vi "check_piezo_travel.vi"() -> ()   [LabVIEW 2015]
uses:
  <vilib>/DAQmx/create/channels.llb/DAQmx Create Channel (AO-Voltage-Basic).vi
  <vilib>/DAQmx/configure/timing.llb/DAQmx Timing (Sample Clock).vi
  <resource>/objmgr/daqmx.rc
  <vilib>/DAQmx/write.llb/DAQmx Write (Analog 1D DBL 1Chan NSamp).vi
  <vilib>/Analysis/NI_AALBase.lvlib
  <vilib>/Analysis/3filter.llb/Bessel Filter (DBL).vi
  <vilib>/Analysis/3filter.llb/Filter Passband Type.ctl
panel:
  out "error out 2":errorcluster
  out "error out":errorcluster
  out "AO SampClk.Rate":dbl
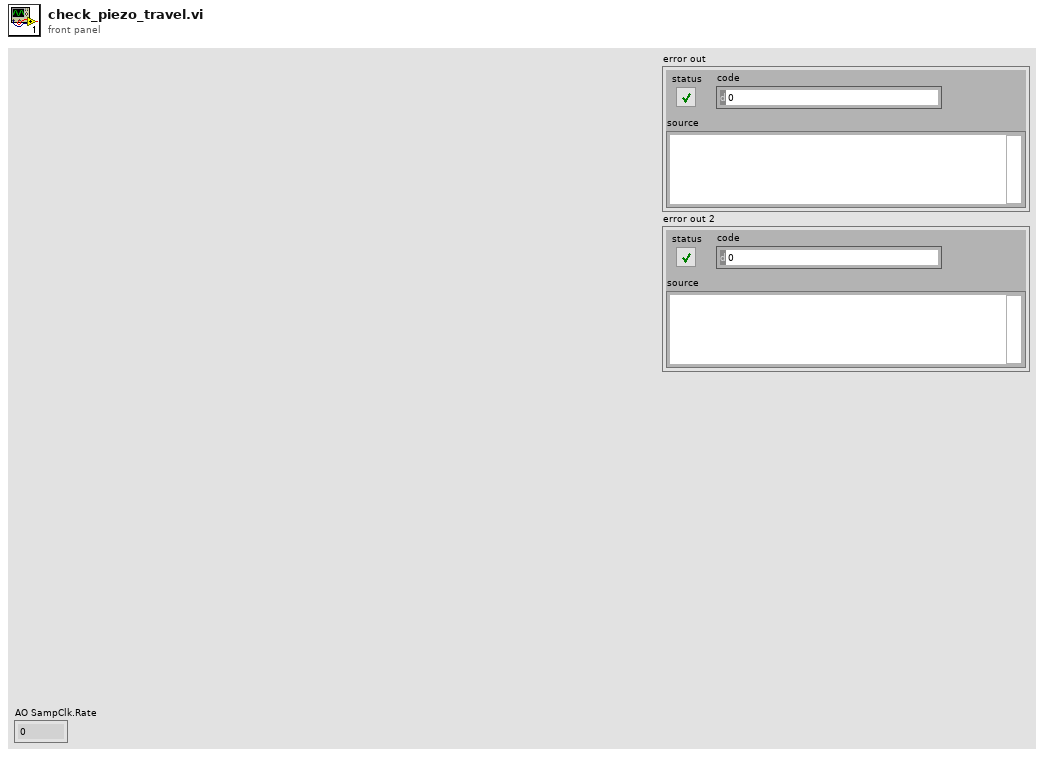
[diagram p1: front panel]
types:
  T1 = typedef "NI_AALBase.lvlib/Filter Passband Type.ctl" = enum32{"Lowpass", "Highpass", "Bandpass", "Bandstop"}
  T2 = typedef "Image Type" = u32
  T3 = typedef "IMAQ Image.ctl" = refnum<image>
  T4 = cluster{"Rows Per Strip":i32, "Photometric":i32, "Compression Type":i32}
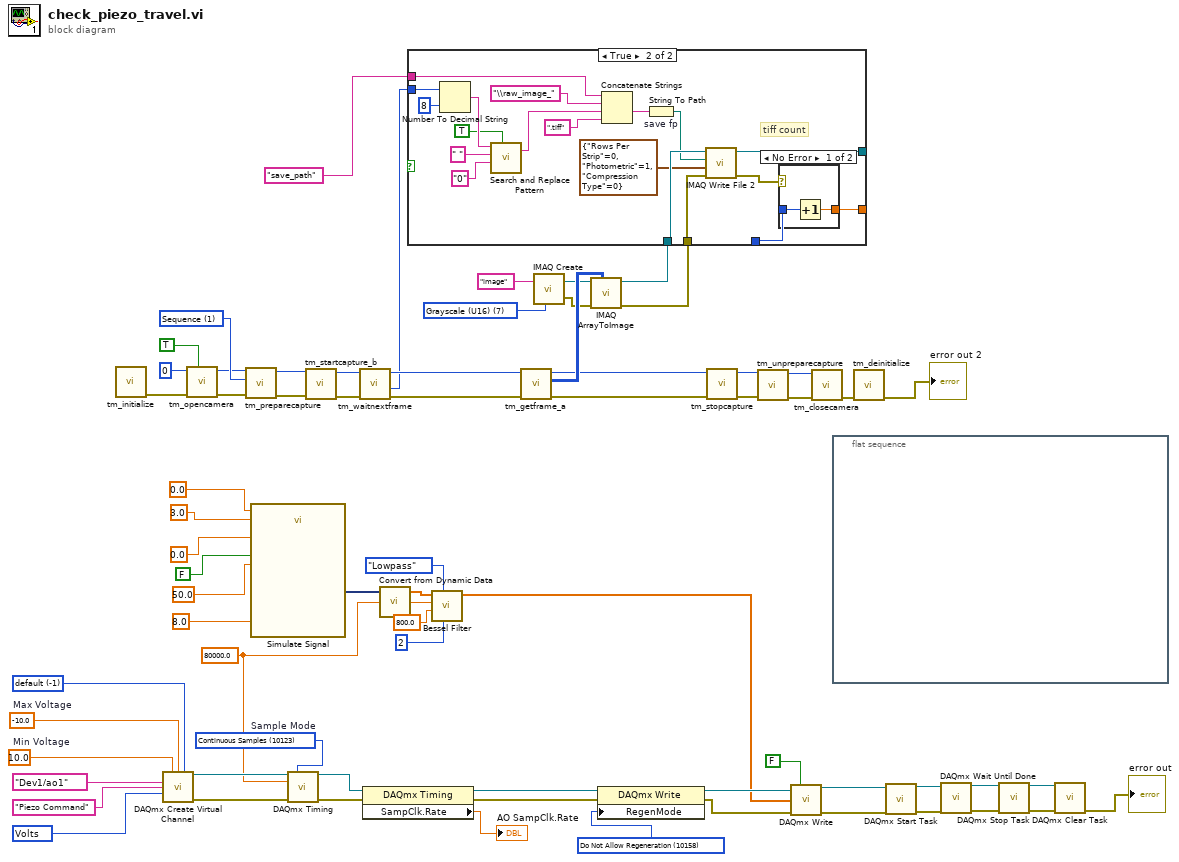
[diagram p0: block diagram]
diagram:
  w10 = 80000.0 ("Rate")
  w34 = 10158 items=["Allow Regeneration"=10097, "Do Not Allow Regeneration"=10158] ("RegenMode")
  w38 = 10123 items=["Finite Samples"=10178, "Continuous Samples"=10123, "Hardware Timed Single Point"=12522]  # Sample Mode
  w45 = -1 items=["default"=-1, "RSE"=10083, "NRSE"=10078, "Differential"=10106, "Pseudodifferential"=12529] ("input terminal configuration")
  w44 = 10348 items=["Volts"=10348, "From Custom Scale"=10065] ("units")
  w41 = 10.0  # Min Voltage
  w42 = -10.0  # Max Voltage
  w57 = T2 7 items=["Grayscale (U8)", "Grayscale (I16)", "Grayscale (SGL)", "Complex (CSG)", "RGB (U32)", "HSL (U32)", "RGB (U64)", "Grayscale (U16)"] ("Image Type")
  w69 = 1 items=["Snap", "Sequence"] ("Capture mode")
  n1 = call <userlib>:"tm_initialize.vi"() -> ("error out"=w68:errorcluster)  [unwired: 8 in, 3 out]
  n2 = call-poly <vilib>:"DAQmx Create Virtual Channel.vi"("maximum value"=w41, "minimum value"=w42, "output terminal configuration"=w45, "physical channels"=tag "Dev1/ao1", "name to assign"="Piezo Command", "units"=w44) -> ("task out"=w39:refnum<k21>, "error out"=w40:errorcluster)  [unwired: 8 in]
  n3 = call <userlib>:"tm_opencamera.vi"("Force Open"=TRUE, "error in (no error)"=w68, "Camera Index"=0) -> ("error out"=w64:errorcluster, "Handle out"=w65:u32)  [unwired: 6 in, 1 out]
  n4 = call <userlib>:"tm_preparecapture.vi"("error in (no error)"=w64, "Capture mode"=w69, "Handle in"=w65) -> ("error out"=w62:errorcluster, "Handle out"=w63:u32)  [unwired: 5 in, 2 out]
  n5 = call "Simulate Signal"("Offset"=0.0, "Duty Cycle (%)"=50.0, "Reset Signal"=FALSE, "Frequency"=3.0, "Amplitude"=8.0, "Phase"=0.0) -> ("Square"=w12:dynamicdata)  [unwired: 8 in, 1 out]
  n6 = call-poly <vilib>:"DAQmx Timing.vi"("task/channels in"=w39, "sample mode"=w38, "rate"=w10, "error in"=w40) -> ("task out"=w36:refnum<k21>, "error out"=w35:errorcluster)  [unwired: 10 in]
  n7 = call <userlib>:"tm_startcapture_b.vi"("error in (no error)"=w62, "Handle in"=w63) -> ("error out"=w60:errorcluster, "Handle out"=w61:u32)  [unwired: 8 in]
  n8 = call <userlib>:"tm_waitnextframe.vi"("error in (no error)"=w60, "Handle in"=w61) -> ("error out"=w58:errorcluster, "Frame Count"=w50:i32, "Handle out"=w59:u32)  [unwired: 6 in, 1 out]
  n9 = property class="DAQmx Timing"(reference=w36, error in=w35) -> (reference out=w47:refnum<k21>, error out=w48:errorcluster, "SampClk.Rate"=→"AO SampClk.Rate":dbl)
  n10 = call "Convert from Dynamic Data"("Dynamic Data Type"=w12) -> ("Array"=w11:dbl[])  [unwired: 3 in]
  n11 = call-poly <vilib>:"Bessel Filter.vi"("order"=2, "filter type"=Filter_Passband_Type."Lowpass", "high cutoff freq: fh"=800.0, "sampling freq: fs"=w10, "X"=w11) -> ("Filtered X"=w2:dbl[])  [unwired: 3 in, 1 out]
  n12 = call <userlib>:"tm_getframe_a.vi"("error in (no error)"=w58, "Handle in"=w59) -> ("error out"=w27:errorcluster, "Data 16"=w55:u16[][], "Handle out"=w28:u32)  [unwired: 5 in, 2 out]
  n13 = call "IMAQ Create"("Image Name"="image", "Image Type"=w57) -> ("New Image"=w53:T3, "error out"=w52:errorcluster)  [unwired: 3 in]
  n14 = call "IMAQ ArrayToImage"("Image Pixels (U16)"=w55, "error in (no error)"=w52, "Image"=w53) -> ("error out"=w51:errorcluster, "Image Out"=w54:T3)  [unwired: 7 in]
  n15 = case shown="True" {
    selector: _ -> [_ _]
    tunnel: w54 -> [w71 w90]
    tunnel: [w71 w88] -> _
    tunnel: "save_path" -> [_ w76]
    tunnel: w50 -> [_ w77]
    tunnel: [w70 w74] -> _
    tunnel: _ -> [w70 w75]
    tunnel: w51 -> [_ w72]
    frame False {
    }
    frame True {
      # "tiff count"
      n16 = Number To Decimal String(number=w77, width (-)=i16 8) -> (decimal integer string=w86:string)
      n17 = call <vilib>:"Search and Replace Pattern.vi"("string"=w86, "regular expression (\"\")"=" " ("regular expression (\"\")"), "replace string (\"\")"="0" ("replace string (\"\")"), "replace all? (F)"=TRUE) -> ("result string"=w87:string)  [unwired: 1 in, 1 out]
      n18 = Concatenate Strings(w76, "\\raw_image_" ("string"), w87, ".tiff" ("string")) -> (w80:string)
      n19 = String To Path "save fp"(string=w80) -> (path=w78:path)
      n20 = call-poly "IMAQ Write File 2"("error in (no error)"=w72, "TIFF Options"=T4 {"Rows Per Strip"=0, "Photometric"=1, "Compression Type"=0}, "File Path"=w78, "Image"=w90) -> ("error out"=w73:errorcluster, "Image Out (duplicate)"=w88:T3)  [unwired: 6 in]
      n21 = case shown="No Error" w73 {
        tunnel: w75 -> [w92 w93]
        tunnel: [w91 w93] -> w74
        frame No Error {
          n22 = Increment(x=w92) -> (x+1=w91:dbl)
        }
        frame Error {
        }
      }
    }
  }
  n23 = property class="DAQmx Write"(reference=w47, error in=w48, "RegenMode"=w34) -> (reference out=w16:refnum<k21>, error out=w15:errorcluster)
  n24 = call <userlib>:"tm_stopcapture.vi"("error in (no error)"=w27, "Handle in"=w28) -> ("error out"=w32:errorcluster, "Handle out"=w33:u32)  [unwired: 8 in]
  n25 = call <userlib>:"tm_unpreparecapture.vi"("error in (no error)"=w32, "Handle in"=w33) -> ("error out"=w29:errorcluster, "Handle out"=w30:u32)  [unwired: 8 in]
  n26 = call-poly <vilib>:"DAQmx Write.vi"("task/channels in"=w16, "auto start"=FALSE, "data"=w2, "error in"=w15) -> ("task out"=w20:refnum<k21>, "error out"=w19:errorcluster)  [unwired: 9 in, 1 out]
  n27 = call <userlib>:"tm_closecamera.vi"("error in (no error)"=w29, "Handle in"=w30) -> ("error out"=w31:errorcluster)  [unwired: 9 in]
  n28 = flat-sequence {
    frame #0 {
    }
  }
  n29 = call <userlib>:"tm_deinitialize.vi"("error in (no error)"=w31) -> ("error out"=→"error out 2":errorcluster)  [unwired: 10 in]
  n30 = call <vilib>:"DAQmx Start Task.vi"("task/channels in"=w20, "error in"=w19) -> ("task out"=w22:refnum<k21>, "error out"=w21:errorcluster)  [unwired: 12 in]
  n31 = call <vilib>:"DAQmx Wait Until Done.vi"("task/channels in"=w22, "error in"=w21) -> ("task out"=w26:refnum<k21>, "error out"=w25:errorcluster)  [unwired: 12 in]
  n32 = call <vilib>:"DAQmx Stop Task.vi"("task/channels in"=w26, "error in"=w25) -> ("task out"=w24:refnum<k21>, "error out"=w23:errorcluster)  [unwired: 12 in]
  n33 = call <vilib>:"DAQmx Clear Task.vi"("task in"=w24, "error in"=w23) -> ("error out"=→"error out":errorcluster)  [unwired: 13 in]
